vi "Close Device Comm.vi"(0 "Device ID":T1(ring), 11 "error in":errorcluster) -> (4 "Device ID Out":T1(ring), 15 "error out":errorcluster)   [LabVIEW 2010]
doc: "This VI first stops the transfer area which is where the Robo Interface writes data to be read and reads data to be written. Then, it stops the USB or Serial communication between your computer and the Robo Interface."
uses:
  Robo Interface.dll
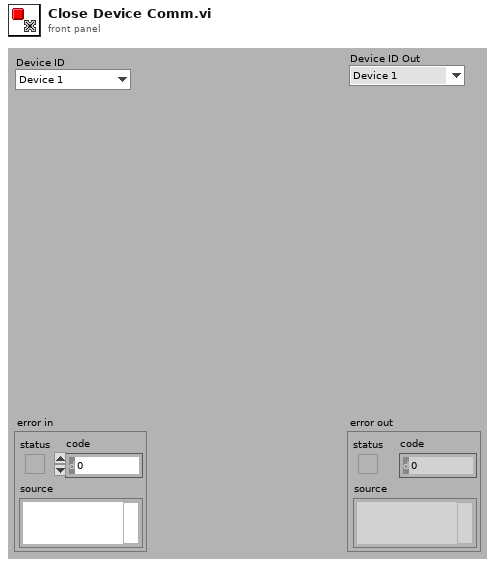
[diagram p1: front panel]
types:
  T1 = enum16{"Device 1", "Device 2", "Device 3", "Device 4", "Device 5", "Device 6", "Device 7", "Device 8"}
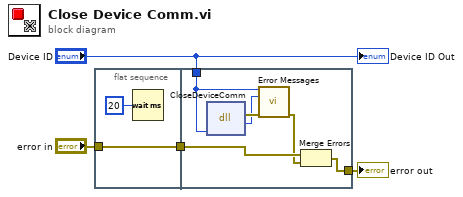
[diagram p0: block diagram]
diagram:
  n1 = flat-sequence {
    tunnel: "error in" -> [w6]
    tunnel: [w6] -> w1
    tunnel: [w9] -> w3
    tunnel: w1 -> [w11]
    tunnel: "Device ID" -> [w7]
    frame #0 {
      n2 = Wait (ms)(milliseconds to wait=u32 20) -> ()  [unwired: 1 out]
    }
    frame #1 {
      n3 = dll-call lib="D:/Aron/LabVIEW-Programmierung/a.F.b.u.s.A/robo_interface_distribute/Robo Interface/Advanced/Robo Interface.dll" fn="CloseDeviceComm"("Device_ID"=w7) -> (error out=w12:errorcluster, "return type"=w8:i32)  [unwired: 3 in, 2 out]
      n4 = call "Error Messages.vi"("Device ID"=w7, "Error Code"=w8, "error in (no error)"=w12) -> ("error out"=w10:errorcluster)  [unwired: 12 out]
      n5 = Merge Errors(w11, w10) -> (w9:errorcluster)
    }
  }
  "error out" <- w3
  "Device ID Out" <- "Device ID"
